vi "Initialize.vi"(8 "error in":errorcluster, 10 "shared resources":refnum<class "Shared Resources.lvclass">, 11 "Ballard ARINC-429 Tx Execution Unit in":refnum<class "Tx Scheduled Labels Execution Unit.lvclass">) -> (0 "error out":errorcluster, 3 "Ballard ARINC-429 Tx Execution Unit out":refnum<class "Tx Scheduled Labels Execution Unit.lvclass">)   [LabVIEW 2020, in "Ballard ARINC 429 Engine.lvlib" / "Implementation.lvlib" / "Tx Scheduled Labels Execution Unit.lvclass"]
uses:
  Tx Scheduled Labels Execution Unit.lvclass
  <instrlib>/BTI429Lib/BTI429LV.lvlib
  Custom Device/Custom Device.lvlib
  Execution Unit/Execution Unit.lvclass
  Shared Resources/Shared Resources.lvclass
  C:/Git/niveristand-ballard-arinc429-custom-device/Source/Custom Device Support/Engine/Implementation/Execution Unit/Execution Unit.lvclass
  C:/Git/niveristand-ballard-arinc429-custom-device/Source/Custom Device Support/Engine/Interfaces/Execution Unit/Execution Unit.lvclass
  C:/Git/niveristand-ballard-arinc429-custom-device/Source/Custom Device Support/Engine/Implementation/Tx Scheduled Labels Execution Unit/Tx Scheduled Labels Execution Unit.lvclass
  Interfaces/Shared Resources/Shared Resources.lvclass
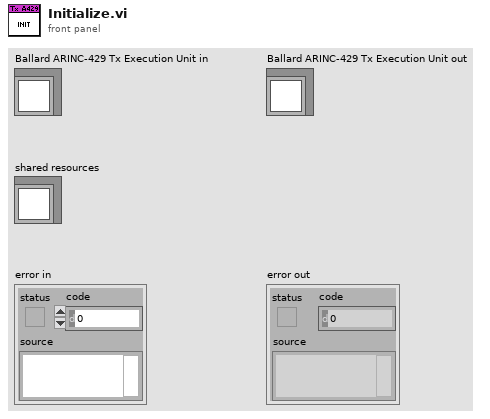
[diagram p1: front panel]
types:
  T1 = typedef "Ballard ARINC 429 Engine.lvlib/Custom Device.lvlib/Hardware Handles.ctl" = cluster{"core handle":u64, "core reader handle":u64, "channel handles":u64[]}
  T2 = typedef "RT Hardware Channel Settings.ctl" = cluster{"channel #":u16, "channel handle":u64, "labels settings for RT":T3[]}
  T3 = typedef "RT Label Settings.ctl" = cluster{"Name":string, "xmlName":string, "label":T4, "transfer period":u32, "SDI_Enabled":bool, "SDI":u8, "parameter driver data":T5, "transfer type":T11, "has timestamp?":bool, "Label Disable/Trigger Channel Reference":T10, "Message Handle":u64, "Initialized?":bool, "Word Initial Raw Value":u32, "Label Timestamp Channel Data Reference":T9, "disabled":bool}
  T4 = typedef "Label.ctl" = u8
  T5 = typedef "RT Parameters.ctl" = cluster{"parameter definitions":T6[], "Rx block data refs":T8[], "Rx values":dbl[], "Tx parameter refs":T10[]}
  T6 = typedef "Parameter Definition.ctl" = cluster{"start index":i32, "size":i32, "encoding":T7, "signed":bool, "scale multiplier":dbl, "scale offset":dbl}
  T7 = typedef "Encoding and Decoding.lvlib/Encoding.ctl" = enum16{"BNR", "BCD", "Discrete"}
  T8 = typedef "Custom Device API.lvlib/Block Data Reference.ctl" = cluster{"Data Reference":T9, "Offset":u64, "Length":u64}
  T9 = typedef "Custom Device API.lvlib/Data Reference.ctl" = i32
  T10 = typedef "Custom Device API.lvlib/Custom Device Item Ref.ctl" = u64
  T11 = typedef "Transfer Type.ctl" = enum16{"Scheduled", "Acyclic", "Block", "Strobe"}
  T12 = typedef "Map of Values Indexes to Channel and Label Indexes.ctl" = map{i32, cluster{"channel index":i32, "label index":i32, "group values start index":i32, "values in group":i32}}
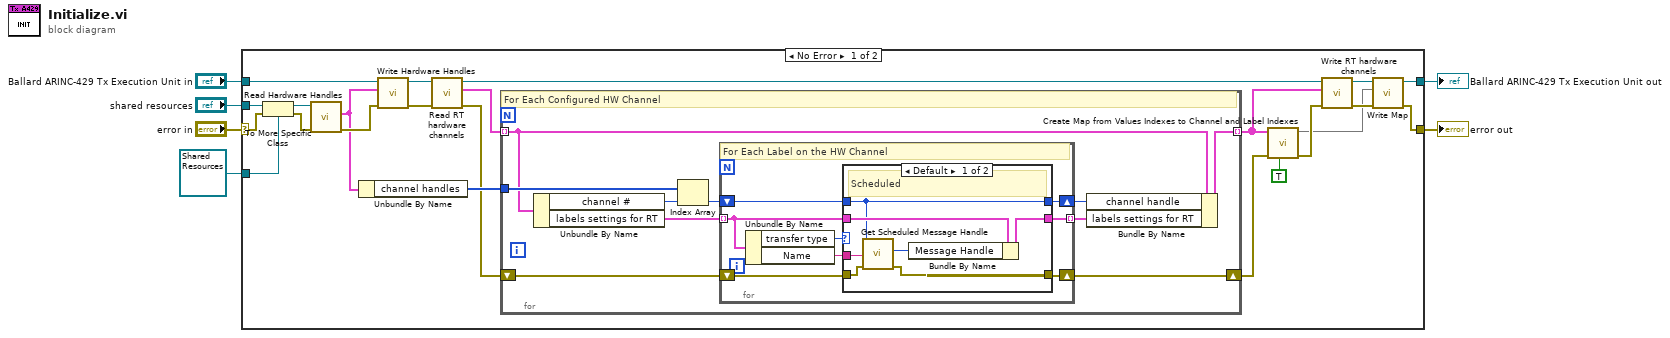
[diagram p0: block diagram]
diagram:
  n1 = case shown="No Error" "error in" {
    selector: "error in" -> [w12 w58]
    tunnel: "Ballard ARINC-429 Tx Execution Unit in" -> [w16 w59]
    tunnel: [w20 w59] -> w5
    tunnel: [w19 w58] -> w3
    tunnel: "shared resources" -> [w10 _]
    tunnel: refnum<class "Shared Resources.lvclass"> refnum ("Ballard ARINC-429 shared resources in") -> [w9 _]
    frame No Error {
      n2 = To More Specific Class(target class=w9, reference=w10, error in=w12) -> (specific class reference=w8:refnum<class "Shared Resources.lvclass">, error out=w11:errorcluster)
      n3 = call "Read Hardware Handles.vi"("error in"=w11, "Ballard ARINC-429 shared resources in"=w8) -> ("error out"=w17:errorcluster, "hardware handles"=w14:T1)  [unwired: 7 in, 1 out]
      n4 = Unbundle By Name(w14) -> ("channel handles"=w29:u64[])
      n5 = call "Write Hardware Handles.vi"("error in"=w17, "hardware handles"=w14, "Ballard ARINC-429 Execution Unit in"=w16) -> ("error out"=w13:errorcluster, "Ballard ARINC-429 Execution Unit out"=w15:refnum<class "Tx Scheduled Labels Execution Unit.lvclass">)  [unwired: 7 in]
      n6 = call "Read RT hardware channels.vi"("error in"=w13, "Ballard ARINC-429 Tx Execution Unit in"=w15) -> ("error out"=w26:errorcluster, "RT hardware channels"=w28:T2[], "Ballard ARINC-429 Tx Execution Unit out"=w27:refnum<class "Tx Scheduled Labels Execution Unit.lvclass">)  [unwired: 7 in]
      n7 = for {
        shift-right: [w30] -> w24
        shift-left: w26 -> [w35]
        tunnel: w28 -> [w34] mode=indexing
        tunnel: w29 -> [w38]
        tunnel: [w31] -> w25 mode=indexing
        # "For Each Configured HW Channel"
        n8 = Unbundle By Name(w34) -> ("channel #"=w39:u16, "labels settings for RT"=w36:T3[])
        n9 = Index Array(array=w38, index=w39) -> (element=w37:u64)
        n10 = for {
          tunnel: w36 -> [w42] mode=indexing
          shift-right: [w43] -> w30
          shift-left: w35 -> [w44]
          tunnel: [w41] -> w33 mode=indexing
          shift-right: [w40] -> w32
          shift-left: w37 -> [w46]
          # "For Each Label on the HW Channel"
          n11 = Unbundle By Name(w42) -> ("transfer type"=w47:T11, "Name"=w45:string)
          n12 = case shown="Default" w47 {
            tunnel: w46 -> [w48 w55]
            tunnel: w45 -> [w54 _]
            tunnel: w44 -> [w53 w57]
            tunnel: [w52 w57] -> w43
            tunnel: w42 -> [w50 w56]
            tunnel: [w49 w56] -> w41
            tunnel: [w48 w55] -> w40
            frame Default {
              # "Scheduled"
              n13 = call <instrlib>:"Get Scheduled Message Handle.vi"("error in (no error)"=w53, "message name"=w54, "channel handle in"=w48) -> ("error out"=w52:errorcluster, "message handle out"=w51:u64)  [unwired: 6 in, 1 out]
              n14 = Bundle By Name(cluster=w50, "Message Handle"=w51) -> (w49:T3)
            }
            frame "Acyclic" {
            }
          }
        }
        n15 = Bundle By Name(cluster=w34, "channel handle"=w32, "labels settings for RT"=w33) -> (w31:T2)
      }
      n16 = call "Create Map from Values Indexes to Channel and Label Indexes.vi"("disable channel included in group"=TRUE, "error in"=w24, "RT hardware channels"=w25) -> ("error out"=w23:errorcluster, "map from values index to RT info indexes"=w18:T12)  [unwired: 7 in]
      n17 = call "Write RT hardware channels.vi"("error in"=w23, "RT hardware channels"=w25, "Ballard ARINC-429 Tx Execution Unit in"=w27) -> ("error out"=w22:errorcluster, "Ballard ARINC-429 Tx Execution Unit out"=w21:refnum<class "Tx Scheduled Labels Execution Unit.lvclass">)  [unwired: 7 in]
      n18 = call "Write Map.vi"("error in"=w22, "map from values indexes to RT info indexes"=w18, "Ballard ARINC-429 Tx Execution Unit in"=w21) -> ("error out"=w19:errorcluster, "Ballard ARINC-429 Tx Execution Unit out"=w20:refnum<class "Tx Scheduled Labels Execution Unit.lvclass">)  [unwired: 7 in]
    }
    frame Error {
    }
  }
  "error out" <- w3
  "Ballard ARINC-429 Tx Execution Unit out" <- w5
